vi "Temprature.vi"(8 "error in (no error)":errorcluster, 11 "LINX Resource in":T1) -> (0 "error out":errorcluster, 1 "Voltage":dbl, 2 "LINX Resource out":T1, 3 "Temp":dbl)   [LabVIEW 2020]
uses:
  <vilib>/MakerHub/LINX/Private/Type Defs/LINX Ref.ctl
  <vilib>/MakerHub/LINX/Private/Type Defs/Platform.ctl
  <vilib>/MakerHub/LINX/Private/Type Defs/Interface.ctl
  <vilib>/MakerHub/LINX/Private/Device/Type Defs/LINX Device Config.ctl
  <vilib>/MakerHub/LINX/Private/Device/Type Defs/TCP Config.ctl
  <vilib>/MakerHub/LINX/Private/Device/Type Defs/Channels.ctl
  <vilib>/MakerHub/LINX/Public/Peripherals/Analog/Analog Read 1 Chan.vi
  <vilib>/MakerHub/LINX/Public/Peripherals/Digital/Digital Write 1 Chan.vi
  <vilib>/MakerHub/LINX/Public/Peripherals/Analog/Analog Read N Chans.vi
  <vilib>/MakerHub/LINX/Public/Peripherals/Digital/Digital Write N Chans.vi
  <vilib>/MakerHub/LINX/Private/Local IO/LinxAnalogRead.vi
  <vilib>/MakerHub/LINX/Public/Utilities/Check Channel.vi
  <vilib>/MakerHub/LINX/Private/Local IO/LinxDigitalWrite.vi
  <vilib>/MakerHub/LINX/Private/Utilties/Generate Error.vi
  <vilib>/MakerHub/LINX/LMH-LINX.lvlib
  <vilib>/MakerHub/LINX/Private/Device/Device.lvlib
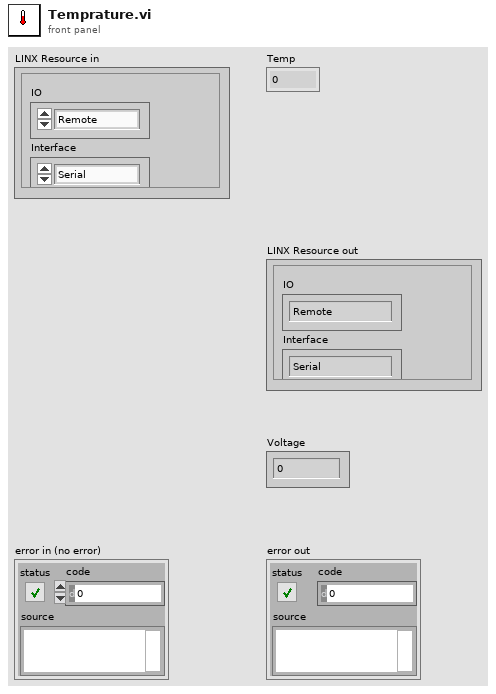
[diagram p1: front panel]
types:
  T1 = typedef "LMH-LINX.lvlib/LINX Ref.ctl" = cluster{"IO":T2, "Interface":T3, "LINX Device Config":T4}
  T2 = typedef "LMH-LINX.lvlib/Platform.ctl" = enum16{"Remote", "Local"}
  T3 = typedef "LMH-LINX.lvlib/Interface.ctl" = enum16{"Serial", "TCP"}
  T4 = typedef "LMH-LINX.lvlib/Device.lvlib/LINX Device Config.ctl" = cluster{"Interface":T3, "COM Port":refnum<visa-resource-name>, "TCP Configuration":T5, "Device Family":u8, "Device ID":u8, "Device Name":string, "TCP Ref":refnum<k5>, "Channels":T6}
  T5 = typedef "LMH-LINX.lvlib/Device.lvlib/TCP Config.ctl" = cluster{"IP Address":string, "Port":u16}
  T6 = typedef "LMH-LINX.lvlib/Channels.ctl" = cluster{"DI":u8[], "DO":u8[], "AI":u8[], "AO":u8[], "PWM":u8[], "QE":u8[], "UART":u8[], "I2C 2":u8[], "SPI":u8[], "CAN":u8[], "Servo":u8[], "AI Ref (V)":dbl, "AI Resolution (Bits)":u8, "AO Ref (V)":dbl, "AO Resolution (Bits)":u8}
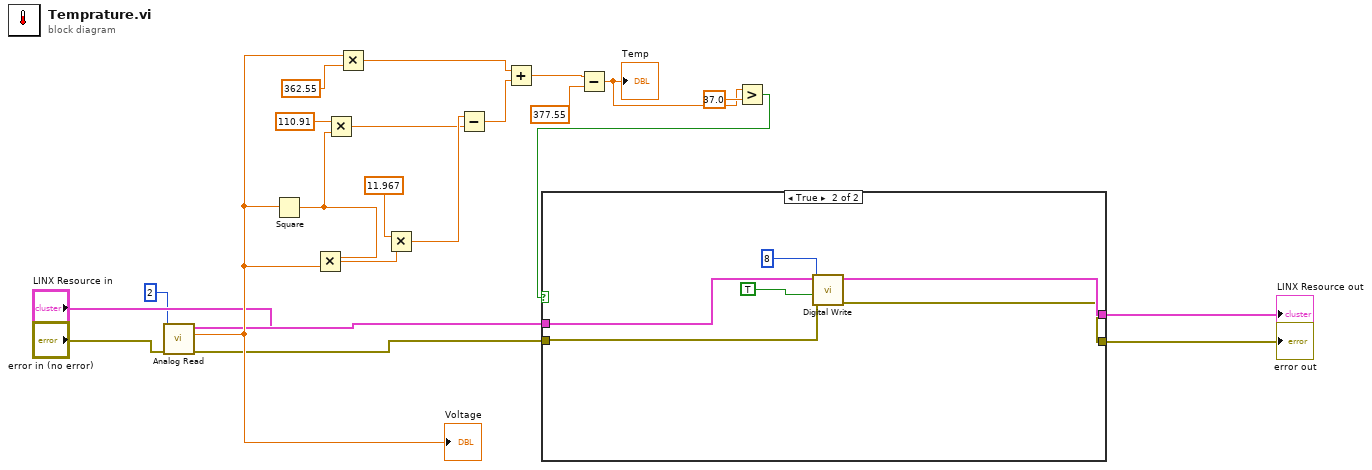
[diagram p0: block diagram]
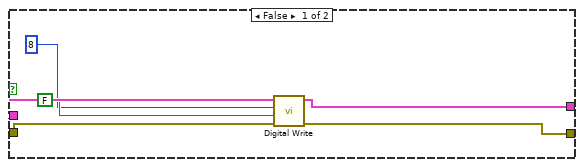
[diagram p2: hidden frame]
diagram:
  n1 = call-poly <vilib>:"Analog Read.vi"("Error In"="error in (no error)", "Analog Channel"=u8 2, "LINX Resource"="LINX Resource in") -> ("Error Out"=w5:errorcluster, "Voltage"=w12:dbl, "LINX Resource"=w4:T1)  [unwired: 5 in, 1 out]
  "Voltage" <- w12
  n2 = Square(x=w12) -> (x^2=w8:dbl)
  n3 = Multiply(x=w8, y=w12) -> (x*y=w7:dbl)
  n4 = Multiply(x=110.91, y=w8) -> (x*y=w10:dbl)
  n5 = Multiply(x=w12, y=362.55) -> (x*y=w14:dbl)
  n6 = Multiply(x=11.967, y=w7) -> (x*y=w11:dbl)
  n7 = Subtract(x=w11, y=w10) -> (x-y=w15:dbl)
  n8 = Add(x=w14, y=w15) -> (x+y=w16:dbl)
  n9 = Subtract(x=w16, y=377.55) -> (x-y=w18:dbl)
  "Temp" <- w18
  n10 = Greater?(x=w18, y=37.0) -> (0:w20:bool)
  n11 = case shown="True" w20 {
    tunnel: w4 -> [w28 w33]
    tunnel: w5 -> [w27 w32]
    tunnel: [w24 w30] -> w21
    tunnel: [w23 w29] -> w22
    frame False {
      n12 = call-poly <vilib>:"Digital Write.vi"("Error In"=w27, "Output Value"=FALSE, "DO Channel"=u8 8, "LINX Resource"=w28) -> ("Error Out"=w23:errorcluster, "LINX Resource"=w24:T1)  [unwired: 6 in]
    }
    frame True {
      n13 = call-poly <vilib>:"Digital Write.vi"("Error In"=w32, "Output Value"=TRUE, "DO Channel"=u8 8, "LINX Resource"=w33) -> ("Error Out"=w29:errorcluster, "LINX Resource"=w30:T1)  [unwired: 6 in]
    }
  }
  "error out" <- w22
  "LINX Resource out" <- w21
